vi "Autonomous Independent.vi"() -> ()   [LabVIEW 2014]
doc: "This VI is called when autonomous begins, and will automatically be terminated when autonomous ends. You can carry out timed or sensor driven robot movement independently without needing to return to the caller."
uses:
  <vilib>/Rock Robotics/WPI/Joystick/WPI_JoystickGetSetRefNum.vi
  <vilib>/Rock Robotics/Network Tables/SD Write Numeric Array.vi
  <vilib>/Rock Robotics/WPI/RobotDrive/WPI_RobotDriveGetSetRefNum.vi
  <vilib>/Rock Robotics/WPI/RobotDrive/WPI_RobotDriveMecanumDrive_Cartesian.vi
panel:
  out "Current Movement, for debugging":T1 {"Z Joystick Value" scale=-1.0..1.0; "Y Joystick Value" scale=1.0..-1.0; "X Joystick Value" scale=-1.0..1.0}
  in  "Array of robot movements":T2(array[cluster]) {"Z Joystick Value" scale=-1.0..1.0; "Y Joystick Value" scale=1.0..-1.0; "X Joystick Value" scale=-1.0..1.0}
  # "Be sure to right-click and choose Data Operations>>Make Current Value default if you want to save the array values with the VI"
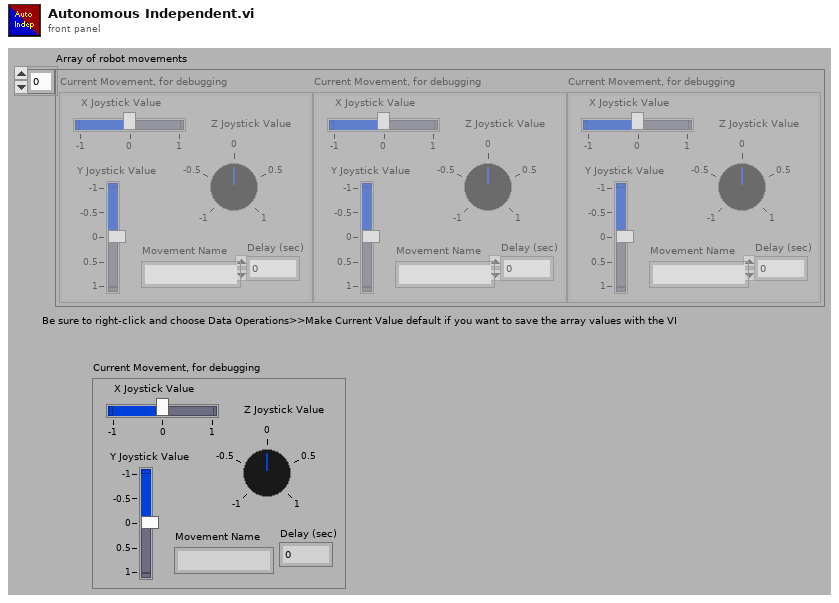
[diagram p1: front panel]
types:
  T1 = cluster{"X Joystick Value":dbl, "Y Joystick Value":dbl, "Z Joystick Value":dbl, "Delay (sec)":dbl, "Movement Name":string}
  T2 = cluster{"X Joystick Value":dbl, "Y Joystick Value":dbl, "Z Joystick Value":dbl, "Delay (sec)":dbl, "Movement Name":string}[]
  T3 = typedef "WPI_JoystickDevRef.ctl" = cluster{"Device":T4}
  T4 = typedef "WPI_JoystickDeviceEnum.ctl" = enum16{"USB 0", "USB 1", "USB 2", "USB 3", "USB 4", "USB 5"}
  T5 = typedef "WPI_RobotDriveDevRef.ctl" = cluster{"DevStatus":errorcluster, "Motors[]":T6[], "Square Inputs":bool, "Max Output":dbl}
  T6 = typedef "WPI_MotorControlDeviceRef.ctl" = cluster{"DeviceStatus":errorcluster, "Type":T7, "PWM":cluster{"Controller":T8, "PWM Channel":T9, "DeadBand":T10}, "CAN":cluster{"Device Number":u8, "Control Mode":T11, "Semaphore":T12, "Max Vout":dbl, "TalonSRX Control Mode":T13}, "Invert":bool, "TransformRef":T14, "InvTransformRef":T14}
  T7 = typedef "WPI_MotorControlType.ctl" = enum16{"PWM", "CAN", "CANTalonSRX"}
  T8 = typedef "FPGA_TypedefDigitalModule.ctl" = enum16{"Controller 1"}
  T9 = typedef "FPGA_DIOPWMChannel.ctl" = enum8{"PWM 0", "PWM 1", "PWM 2", "PWM 3", "PWM 4", "PWM 5", "PWM 6", "PWM 7", "PWM 8", "PWM 9", "PWM MXP 0", "PWM MXP 1", "PWM MXP 2", "PWM MXP 3", "PWM MXP 4", "PWM MXP 5", "PWM MXP 6", "PWM MXP 7", "PWM MXP 8", "PWM MXP 9", "Invalid"}
  T10 = typedef "WPI_PWMDeadband.ctl" = cluster{"Name":string, "maxPositivePwm":i32, "minPositivePwm":i32, "centerPwm":i32, "maxNegativePwm":i32, "minNegativePwm":i32, "angularRange":u16}
  T11 = typedef "WPI_CANJaguar_ControlMode.ctl" = enum8{"Percent VBus", "Current", "Speed", "Position", "Voltage"}
  T12 = typedef "Semaphore RefNum" = refnum<k1>
  T13 = typedef "WPI_CANTalonSRX_APIControlMode.ctl" = enum8{"Percent VBus", "Speed", "Position", "Slave", "Unchanged / Invalid"}
  T14 = typedef "WPI_PWMTransform_ConPane.ctl" = refnum<vi>
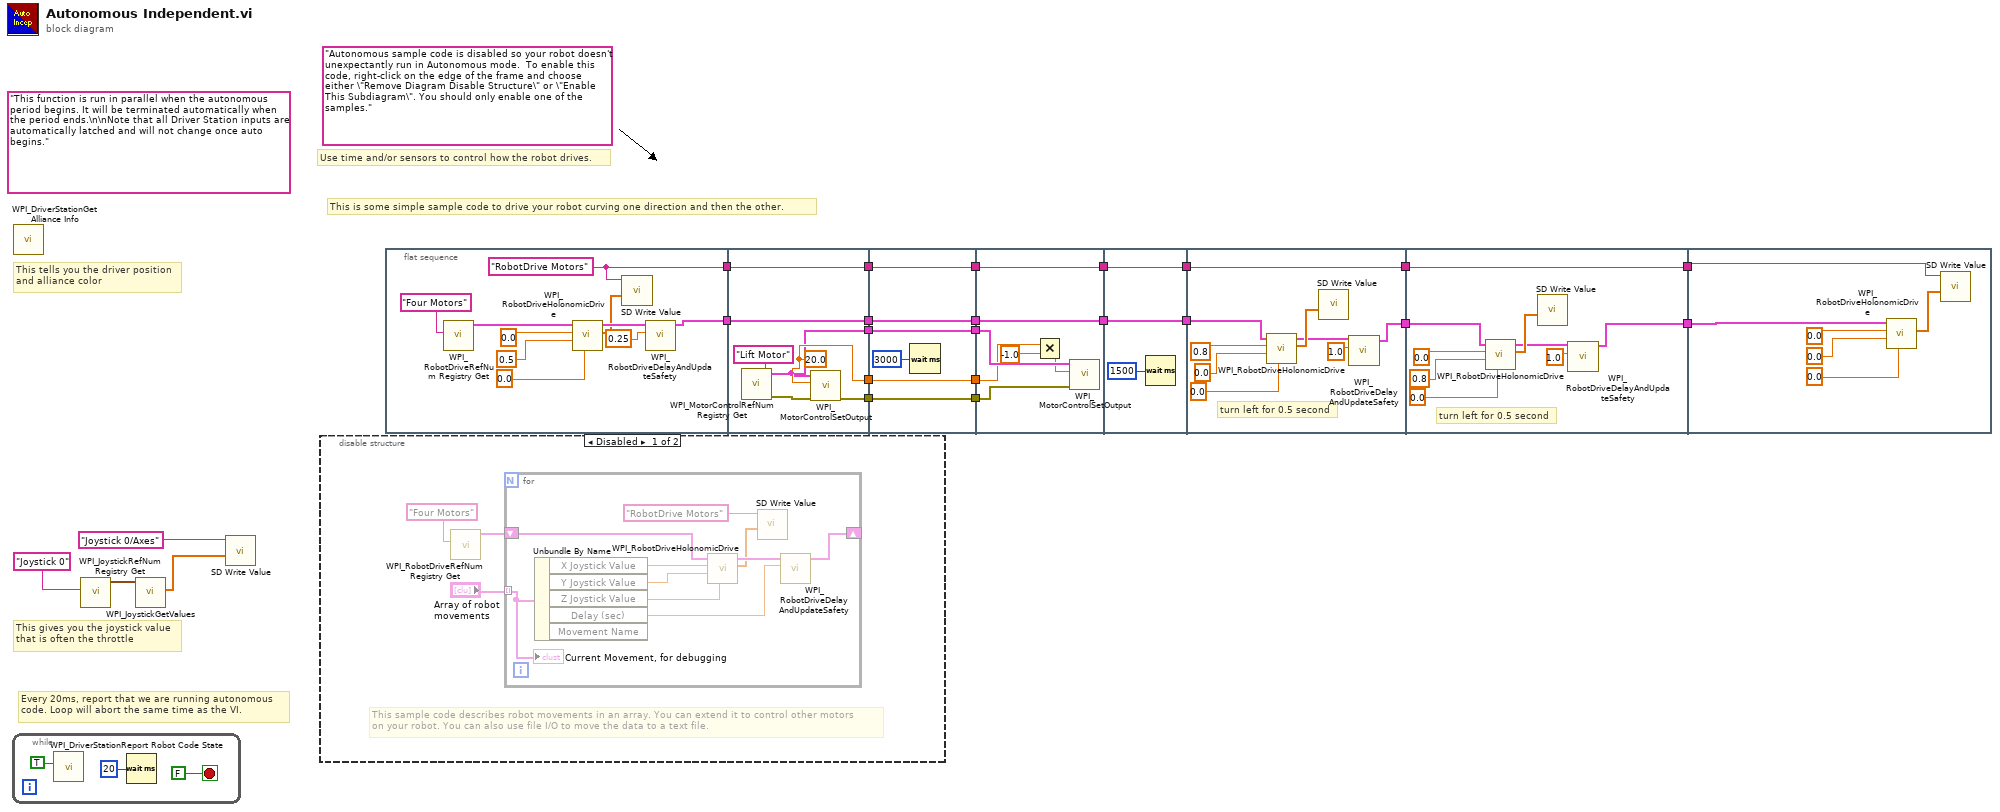
[diagram p0: block diagram]
diagram:
  (unwired) "Autonomous sample code is disabled so your robot doesn't unexpectantly run in Autonomous mode.  To enable this code, right-click on the edge of the frame and choose either \"Remove Diagram Disable Structure\" or \"Enable This Subdiagram\". You should only enable one of the samples."
  (unwired) "This function is run in parallel when the autonomous period begins. It will be terminated automatically when the period ends.\n\nNote that all Driver Station inputs are automatically latched and will not change once auto begins."
  # "This is some simple sample code to drive your robot curving one direction and then the other."
  # "Every 20ms, report that we are running autonomous\ncode. Loop will abort the same time as the VI."
  # "This gives you the joystick value\nthat is often the throttle"
  # "Use time and/or sensors to control how the robot drives."
  # "This tells you the driver position\nand alliance color"
  n1 = while {
    stop <- FALSE stop-if-true
    n2 = call <vilib>:"WPI_DriverStationReport Robot Code State.vi"("Autonomous"=TRUE) -> ()  [unwired: 10 in, 1 out]
    n3 = Wait (ms)(milliseconds to wait=u32 20) -> ()  [unwired: 1 out]
  }
  n4 = call <vilib>:"WPI_DriverStationGet Alliance Info.vi"() -> ()  [unwired: 12 out]
  n5 = call <vilib>:"WPI_JoystickRefNum Registry Get.vi"("refnum name"="Joystick 0") -> ("JoystickDevRef"=w23:T3)  [unwired: 1 in, 9 out]
  n6 = call <vilib>:"WPI_JoystickGetValues.vi"("JoystickDevRef"=w23) -> ("Axes"=w21:dbl[])  [unwired: 6 in, 4 out]
  n7 = call-poly <vilib>:"SD Write Value.vi"("Numeric Array"=w21, "Name"="Joystick 0/Axes") -> ()  [unwired: 8 in, 2 out]
  n8 = disable-structure shown="Disabled" {
    frame Disabled {
      # "This sample code describes robot movements in an array. You can extend it to control other motors\non your robot. You can also use file I/O to move the data to a text file."
      n9 = call <vilib>:"WPI_RobotDriveRefNum Registry Get.vi"("refnum name"="Four Motors") -> ("RobotDriveDevRef"=w29:T5)  [unwired: 1 in, 9 out]
      n10 = for {
        shift-right: [w37] -> _
        shift-left: w29 -> [w38]
        tunnel: "Array of robot movements" -> [w33] mode=indexing
        n11 = Unbundle By Name(w33) -> ("X Joystick Value"=w36:dbl, "Y Joystick Value"=w35:dbl, "Z Joystick Value"=w32:dbl, "Delay (sec)"=w34:dbl)  [unwired: 1 out]
        n12 = call-poly <vilib>:"WPI_RobotDriveHolonomicDrive.vi"("Rotation"=w32, "Y"=w35, "X"=w36, "RobotDriveDevRef"=w38) -> ("Motor Values"=w31:dbl[], "RobotDriveDevRef"=w39:T5)  [unwired: 5 in, 1 out]
        n13 = call-poly <vilib>:"SD Write Value.vi"("Numeric Array"=w31, "Name"="RobotDrive Motors") -> ()  [unwired: 8 in, 2 out]
        n14 = call <vilib>:"WPI_RobotDriveDelayAndUpdateSafety.vi"("Delay (s)"=w34, "RobotDriveDevRef"=w39) -> ("RobotDriveDevRef 2"=w37:T5)  [unwired: 8 in, 1 out]
        "Current Movement, for debugging" <- w33
      }
    }
    frame Enabled {
    }
  }
  n15 = flat-sequence {
    tunnel: [w42] -> w20
    tunnel: [w41] -> w19
    tunnel: w20 -> [w57]
    tunnel: [w57] -> w18
    tunnel: w19 -> [w56]
    tunnel: [w56] -> w17
    tunnel: [w53] -> w14
    tunnel: [w52] -> w11
    tunnel: [w51] -> w10
    tunnel: w18 -> [w63]
    tunnel: [w63] -> w16
    tunnel: w17 -> [w62]
    tunnel: [w62] -> w15
    tunnel: w14 -> [w60]
    tunnel: [w60] -> w13
    tunnel: [w59] -> w12
    tunnel: w11 -> [w59]
    tunnel: w10 -> [w58]
    tunnel: [w58] -> w9
    tunnel: w16 -> [w70]
    tunnel: [w70] -> w8
    tunnel: w15 -> [w69]
    tunnel: [w69] -> w7
    tunnel: w13 -> [w66]
    tunnel: w12 -> [w68]
    tunnel: w9 -> [w67]
    tunnel: w8 -> [w73]
    tunnel: [w73] -> w6
    tunnel: w7 -> [w72]
    tunnel: [w72] -> w5
    tunnel: w6 -> [w75]
    tunnel: w5 -> [w82]
    tunnel: [w82] -> w4
    tunnel: [w74] -> w2
    tunnel: w4 -> [w91]
    tunnel: [w91] -> w3
    tunnel: w2 -> [w84]
    tunnel: [w83] -> w1
    tunnel: w3 -> [w93]
    tunnel: w1 -> [w92]
    frame #0 {
      w41 = "RobotDrive Motors" ("Name")
      n16 = call <vilib>:"WPI_RobotDriveRefNum Registry Get.vi"("refnum name"="Four Motors") -> ("RobotDriveDevRef"=w45:T5)  [unwired: 1 in, 9 out]
      n17 = call-poly <vilib>:"WPI_RobotDriveHolonomicDrive.vi"("Rotation"=0.0, "Y"=0.5 ("X axis value"), "X"=0.0 ("X axis value"), "RobotDriveDevRef"=w45) -> ("Motor Values"=w43:dbl[], "RobotDriveDevRef"=w48:T5)  [unwired: 5 in, 1 out]
      n18 = call-poly <vilib>:"SD Write Value.vi"("Numeric Array"=w43, "Name"=w41) -> ()  [unwired: 8 in, 2 out]
      n19 = call <vilib>:"WPI_RobotDriveDelayAndUpdateSafety.vi"("Delay (s)"=0.25, "RobotDriveDevRef"=w48) -> ("RobotDriveDevRef 2"=w42:T5)  [unwired: 8 in, 1 out]
    }
    frame #1 {
      w53 = 20.0 ("Output")
      n20 = call <vilib>:"WPI_MotorControlRefNum Registry Get.vi"("refnum name"="Lift Motor") -> ("error out"=w54:errorcluster, "MotorControlDevRef"=w52:T6)  [unwired: 9 in]
      n21 = call <vilib>:"WPI_MotorControlSetOutput.vi"("error in (no error)"=w54, "Output"=w53, "MotorControlDevRef"=w52) -> ("error out"=w51:errorcluster)  [unwired: 6 in, 2 out]
    }
    frame #2 {
      n22 = Wait (ms)(milliseconds to wait=u32 3000) -> ()  [unwired: 1 out]
    }
    frame #3 {
      n23 = Multiply(x=w66, y=-1.0) -> (x*y=w64:dbl)
      n24 = call <vilib>:"WPI_MotorControlSetOutput.vi"("error in (no error)"=w67, "Output"=w64, "MotorControlDevRef"=w68) -> ()  [unwired: 6 in, 3 out]
    }
    frame #4 {
      n25 = Wait (ms)(milliseconds to wait=u32 1500) -> ()  [unwired: 1 out]
    }
    frame #5 {
      # "turn left for 0.5 second"
      n26 = call-poly <vilib>:"WPI_RobotDriveHolonomicDrive.vi"("Rotation"=0.0, "Y"=0.0 ("X axis value"), "X"=0.8 ("X axis value"), "RobotDriveDevRef"=w75) -> ("Motor Values"=w81:dbl[], "RobotDriveDevRef"=w78:T5)  [unwired: 5 in, 1 out]
      n27 = call-poly <vilib>:"SD Write Value.vi"("Numeric Array"=w81) -> ()  [unwired: 9 in, 2 out]
      n28 = call <vilib>:"WPI_RobotDriveDelayAndUpdateSafety.vi"("Delay (s)"=1.0, "RobotDriveDevRef"=w78) -> ("RobotDriveDevRef 2"=w74:T5)  [unwired: 8 in, 1 out]
    }
    frame #6 {
      # "turn left for 0.5 second"
      n29 = call-poly <vilib>:"WPI_RobotDriveHolonomicDrive.vi"("Rotation"=0.0, "Y"=0.8 ("X axis value"), "X"=0.0 ("X axis value"), "RobotDriveDevRef"=w84) -> ("Motor Values"=w90:dbl[], "RobotDriveDevRef"=w87:T5)  [unwired: 5 in, 1 out]
      n30 = call-poly <vilib>:"SD Write Value.vi"("Numeric Array"=w90) -> ()  [unwired: 9 in, 2 out]
      n31 = call <vilib>:"WPI_RobotDriveDelayAndUpdateSafety.vi"("Delay (s)"=1.0, "RobotDriveDevRef"=w87) -> ("RobotDriveDevRef 2"=w83:T5)  [unwired: 8 in, 1 out]
    }
    frame #7 {
      n32 = call-poly <vilib>:"WPI_RobotDriveHolonomicDrive.vi"("Rotation"=0.0 ("X axis value"), "Y"=0.0 ("X axis value"), "X"=0.0 ("X axis value"), "RobotDriveDevRef"=w92) -> ("Motor Values"=w97:dbl[])  [unwired: 5 in, 2 out]
      n33 = call-poly <vilib>:"SD Write Value.vi"("Numeric Array"=w97, "Name"=w93) -> ()  [unwired: 8 in, 2 out]
    }
  }
